vi "SetControllerEnqueuer.vi"(8 "error in (no error)":errorcluster, 10 "Controller Enqueuer":refnum<class "Message Enqueuer.lvclass">, 11 "Device in":refnum<class "Device.lvclass">) -> (0 "error out":errorcluster, 2 "Controller Enqueue Out":refnum<class "Message Enqueuer.lvclass">, 3 "Device out":refnum<class "Device.lvclass">)   [LabVIEW 2020, in "Device.lvlib" / "Device.lvclass"]
uses:
  Device.lvclass
  <vilib>/ActorFramework/Message Enqueuer/Message Enqueuer.lvclass
  Device.lvclass/Device.ctl
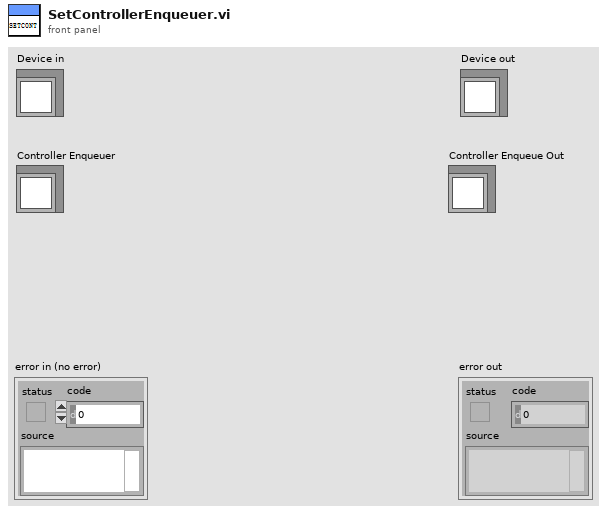
[diagram p1: front panel]
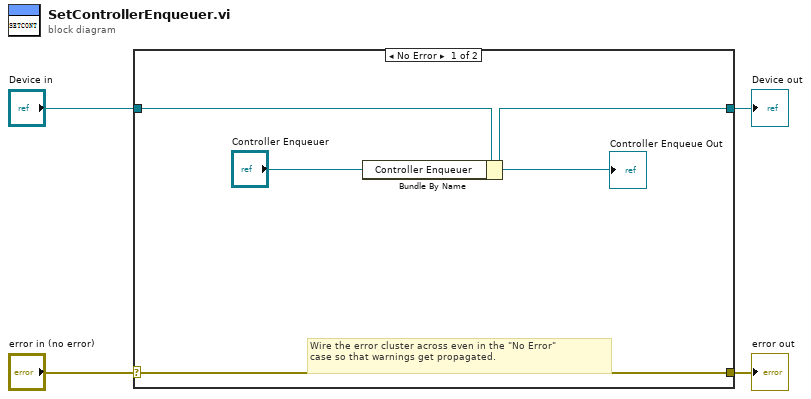
[diagram p0: block diagram]
diagram:
  n1 = case shown="No Error" "error in (no error)" {
    selector: "error in (no error)" -> [w7 w10]
    tunnel: [w7 w10] -> w3
    tunnel: [w6 w9] -> w1
    tunnel: "Device in" -> [w8 w9]
    frame No Error {
      # "Wire the error cluster across even in the \"No Error\"\ncase so that warnings get propagated."
      n2 = Bundle By Name(cluster=w8, "Controller Enqueuer"="Controller Enqueuer") -> (w6:refnum<class "Device.lvclass">)
      "Controller Enqueue Out" <- "Controller Enqueuer"
    }
    frame Error {
    }
  }
  "error out" <- w3
  "Device out" <- w1
